vi "parse single action command.vi"(8 "error in":errorcluster, 11 "message data":string) -> (0 "error out":errorcluster, 3 "engine name":string)   [LabVIEW 2014, in "SMSLD TBD execution service.lvlib"]
uses:
  SMSLD TBD execution service.lvlib
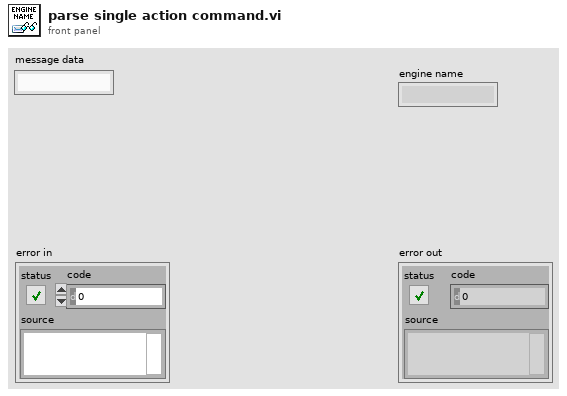
[diagram p1: front panel]
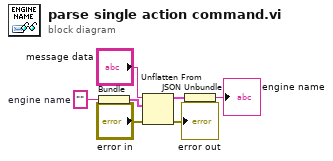
[diagram p0: block diagram]
diagram:
  w2 = ""  # engine name
  n1 = Bundle("engine name"=w2) -> (w4:cluster{"engine name":string})  [unwired: 1 in]
  n2 = Unflatten From JSON(JSON string="message data", type and defaults=w4, error in (no error)="error in") -> (value=w3:cluster{"engine name":string}, error out=→"error out":errorcluster)  [unwired: 4 in]
  n3 = Unbundle(w3) -> ("engine name"=→"engine name":string)
